vi "Call Function with IMAQ Objects.vi"(8 "error in (no error)":errorcluster) -> (0 "error out":errorcluster)   [LabVIEW 2020]
uses:
  G-Embedded-Python-Interpreter-Toolkit/G-Embedded-Python-Interpreter-Toolkit.lvlib
  <vilib>/addons/_JKI Toolkits/Caraya/classes/Test/Test.lvclass
  <vilib>/addons/_JKI Toolkits/Caraya/classes/Assert/Assert.lvclass
  908d8fb0-7b42-46e8-9e96-a0c6d44c2c93.vi
  G-Embedded-Python-Interpreter-Toolkit-IMAQ/G-Embedded-Python-Interpreter-Toolkit-IMAQ.lvlib
  <vilib>/addons/_JKI Toolkits/Caraya/classes/Assert/Assert Equal Value and Type_Variant.vi
  <vilib>/addons/_JKI Toolkits/Caraya/classes/Assert/Assert Not Error.vi
panel:
  out "Image":T1(plugin-control)
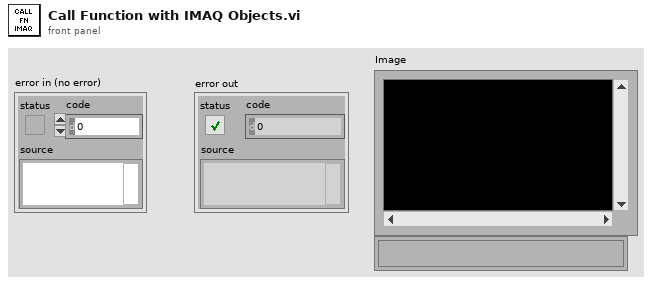
[diagram p1: front panel]
types:
  T1 = typedef "IMAQ Image.ctl" = refnum<image>
  T2 = cluster{"left":i16, "top":i16, "right":i16, "bottom":i16}
  T3 = typedef "Image Type" = u32
  T4 = typedef "imagedata.ctl" = cluster{"image type":i32, "image depth":i32, "image":u8[], "mask":u8[], "colors":u32[], "Rectangle":cluster{"left":i16, "top":i16, "right":i16, "bottom":i16}}
  T5 = typedef "G-Embedded-Python-Interpreter-Toolkit.lvlib/Python Object Reference.ctl" = refnum<k1>
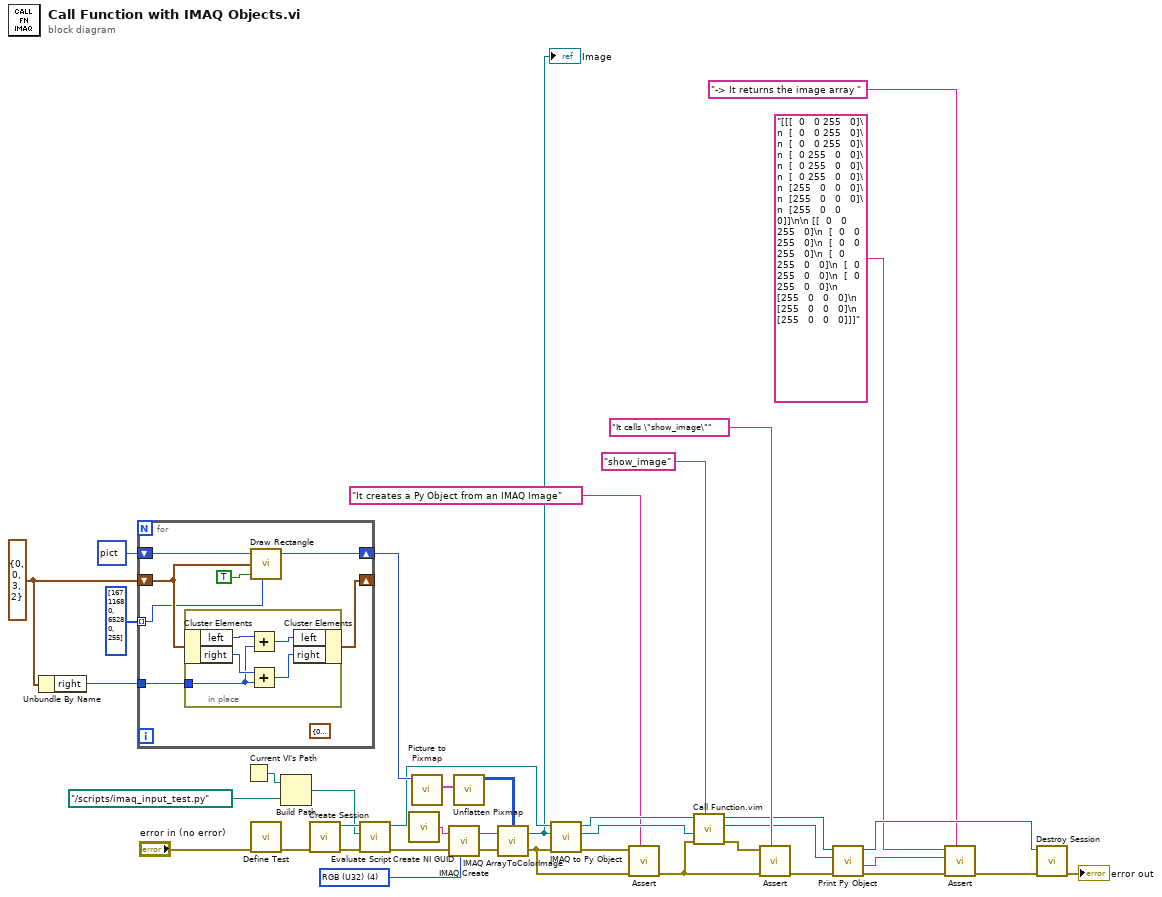
[diagram p0: block diagram]
diagram:
  w17 = T2 {"left"=0, "top"=0, "right"=3, "bottom"=2} ("rect")
  w28 = T3 4 items=["Grayscale (U8)", "Grayscale (I16)", "Grayscale (SGL)", "Complex (CSG)", "RGB (U32)", "HSL (U32)", "RGB (U64)", "Grayscale (U16)"] ("Image Type")
  n1 = Unbundle By Name(w17) -> ("right"=w16:i16)
  n2 = for {
    tunnel: u32[] [16711680, 65280, 255] ("color(black)") -> [w41] mode=indexing
    shift-right: [w46] -> w24
    shift-left: picture data[5B] ("new picture") -> [w45]
    shift-right: [w42] -> _
    shift-left: w17 -> [w44]
    tunnel: w16 -> [w43]
    (unwired) T2 {"left"=0, "top"=0, "right"=0, "bottom"=0} ("rect")
    n3 = in-place {
      in-place-border: w43 -> [w49]
      n4 = in-place-cluster #1(w44) -> ("left"=w52:i16, "right"=w50:i16)
      n5 = Add(x=w52, y=w49) -> (x+y=w51:i16)
      n6 = Add(x=w50, y=w49) -> (x+y=w48:i16)
      n7 = in-place-cluster #1("left"=w51, "right"=w48) -> (w42:T2)
    }
    n8 = call <vilib>:"Draw Rectangle.vi"("picture"=w45, "rect"=w44, "fill?(F)"=TRUE, "color(black)"=w41) -> ("new picture"=w46:picture)  [unwired: 5 in]
  }
  n9 = Current VI's Path() -> (path=w36:path)
  n10 = call <vilib>:"Define Test.vi"("error in (no error)"="error in (no error)") -> ("error out"=w40:errorcluster)  [unwired: 10 in]
  n11 = Build Path(base path=w36, name or relative path=path "../scripts/imaq_input_test.py" ("Path")) -> (appended path=w34:path)
  n12 = call "Create Session.vi"("error in (no error)"=w40) -> ("error out"=w33:errorcluster, "Session Handle"=w37:refnum<data-value>)  [unwired: 9 in]
  n13 = call "Evaluate Script.vi"("error in (no error)"=w33, "Script File Path"=w34, "Session Handle in"=w37) -> ("error out"=w22:errorcluster, "Session Handle out"=w20:refnum<data-value>)  [unwired: 7 in]
  n14 = call <vilib>:"Create NI GUID.vi"() -> ("NI GUID"=w27:string)
  n15 = call <vilib>:"Picture to Pixmap.vi"("picture"=w24) -> ("image data"=w23:T4)  [unwired: 9 in, 1 out]
  n16 = call "IMAQ Create"("Image Name"=w27, "Image Type"=w28, "error in (no error)"=w22) -> ("New Image"=w26:T1, "error out"=w21:errorcluster)  [unwired: 2 in]
  n17 = call <vilib>:"Unflatten Pixmap.vi"("image data"=w23) -> ("24-bit pixmap"=w25:u32[][])  [unwired: 4 in, 6 out]
  n18 = call "IMAQ ArrayToColorImage"("Image Pixels (U32)"=w25, "Image"=w26, "error in (no error)"=w21) -> ("Image Out"=w18:T1, "error out"=w3:errorcluster)  [unwired: 2 in]
  "Image" <- w18
  n19 = call "IMAQ to Py Object.vi"("error in (no error)"=w3, "Image In"=w18, "Session Handle in"=w20) -> ("error out"=w4:errorcluster, "Python Object Refnum"=w15:T5, "Session Handle out"=w19:refnum<data-value>)  [unwired: 6 in]
  n20 = call-poly <vilib>:"Assert.vi"("Label"="It creates a Py Object from an IMAQ Image", "error in (no error)"=w3, "Not Error?"=w4) -> ("error out"=w2:errorcluster)  [unwired: 8 in]
  n21 = call "Call Function.vim"("Function Name"="show_image", "error in (no error)"=w2, "Arguments in (Default - None)"=w15, "Data Value Reference in"=w19) -> ("error out"=w14:errorcluster, "Returned Python Object Refnum"=w8:T5, "Data Value Reference out"=w13:refnum<data-value>)  [unwired: 5 in]
  n22 = call-poly <vilib>:"Assert.vi"("Label"="It calls \"show_image\"", "error in (no error)"=w2, "Not Error?"=w14) -> ("error out"=w11:errorcluster)  [unwired: 8 in]
  n23 = call "Print Py Object.vi"("error in (no error)"=w11, "Python Object Refnum in"=w8, "Session Handle in"=w13) -> ("error out"=w10:errorcluster, "Print Ouptut"=w6:string, "Session Handle out"=w12:refnum<data-value>)  [unwired: 5 in, 1 out]
  n24 = call-poly <vilib>:"Assert.vi"("Label"="-> It returns the image array ", "error in (no error)"=w10, "Y"=w6, "X"="[[[  0   0 255   0]\n  [  0   0 255   0]\n  [  0   0 255   0]\n  [  0 255   0   0]\n  [  0 255   0   0]\n  [  0 255   0   0]\n  [255   0   0   0]\n  [255   0   0   0]\n  [255   0   0   0]]\n\n [[  0   0 255   0]\n  [  0   0 255   0]\n  [  0   0 255   0]\n  [  0 255   0   0]\n  [  0 255   0   0]\n  [  0 255   0   0]\n  [255   0   0   0]\n  [255   0   0   0]\n  [255   0   0   0]]]" ("Print Ouptut")) -> ("error out"=w9:errorcluster)  [unwired: 7 in]
  n25 = call "Destroy Session.vi"("error in (no error)"=w9, "Session Handle"=w12) -> ("error out"=→"error out":errorcluster)  [unwired: 9 in]
